vi "Calculate Position Orientation.vi"(8 "error in":errorcluster, 10 "Measured Global Positions":refnum<class "Vec3d Class.lvclass">[](array[class]), 11 "Known Local Positions":refnum<class "Vec3d Class.lvclass">[](array[class])) -> (0 "error out":errorcluster, 1 "Residual":dbl, 3 "PositionOrientation":T1)   [LabVIEW 2011]
uses:
  Vec3d Class/Vec3d Class.lvclass
  Type Definitions/Position_Orientation.ctl
  Orient3d Class/Orient3d Class.lvclass
  <vilib>/Analysis/_algsub.llb/Vector Norm Type.ctl
  <vilib>/Analysis/baseanly.llb/Real A x B.vi
  <vilib>/Analysis/_algsub.llb/Real Vector Norm.vi
  <vilib>/Analysis/7linalg.llb/Real Matrix Power.vi
  <vilib>/Analysis/Matrix/Numeric/Add/Add - RM,RM.vi
  <vilib>/Analysis/NI_AALBase.lvlib
  <vilib>/Analysis/NI_AALPro.lvlib
  <vilib>/Analysis/Matrix/NI_Matrix.lvlib
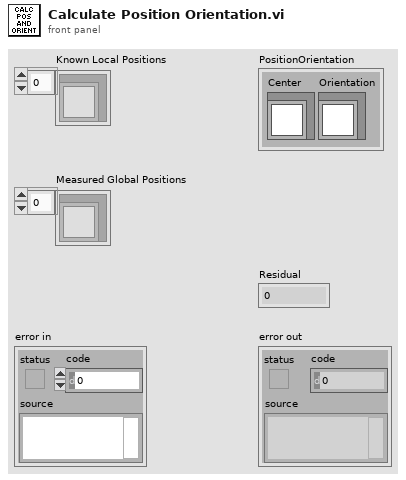
[diagram p1: front panel]
types:
  T1 = typedef "Position_Orientation.ctl" = cluster{"Center":refnum<class "Vec3d Class.lvclass">, "Orientation":refnum<class "Orient3d Class.lvclass">}
  T2 = typedef "NI_AALPro.lvlib/Vector Norm Type.ctl" = u16
  T3 = typedef "NI_Matrix.lvlib/RealMatrix.ctl" = dbl[][]
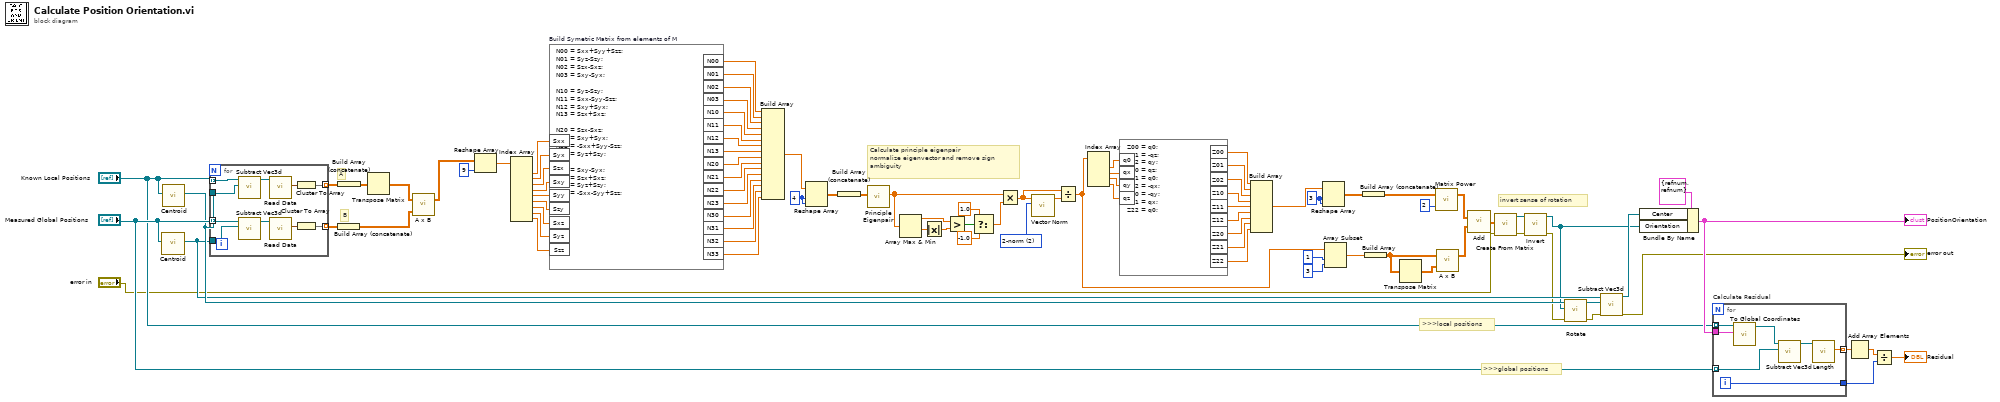
[diagram p0: block diagram]
diagram:
  w11 = 3 ("dimension size")
  w27 = 4 ("dimension size")
  w72 = T2 2 items=["1-norm"=1, "2-norm"=2, "Inf-norm"=3, "-Inf-norm"=4, "User Defined"=5] ("norm type")
  # "invert sense of rotation"
  # ">>>local positions"
  # ">>>global positions"
  # "Calculate principle eigenpair\nnormalize eigenvector and remove sign\nambiguity"
  # "B"
  # "A"
  n1 = call "Centroid.vi"("Points"="Measured Global Positions") -> ("Centroid"=w61:refnum<class "Vec3d Class.lvclass">)  [unwired: 10 in]
  n2 = call "Centroid.vi"("Points"="Known Local Positions") -> ("Centroid"=w62:refnum<class "Vec3d Class.lvclass">)  [unwired: 10 in]
  n3 = for {
    tunnel: "Known Local Positions" -> [w104] mode=indexing
    tunnel: "Measured Global Positions" -> [w102] mode=indexing
    tunnel: w61 -> [w101]
    tunnel: w62 -> [w103]
    tunnel: [w96] -> w86 mode=indexing
    tunnel: [w95] -> w85 mode=indexing
    n4 = call "Subtract Vec3d.vi"("Vec3d in 2"=w103, "Vec3d in 1"=w104) -> ("Vec3d Class out"=w100:refnum<class "Vec3d Class.lvclass">)  [unwired: 8 in, 1 out]
    n5 = call "Subtract Vec3d.vi"("Vec3d in 2"=w101, "Vec3d in 1"=w102) -> ("Vec3d Class out"=w97:refnum<class "Vec3d Class.lvclass">)  [unwired: 8 in, 1 out]
    n6 = call-dynamic "Read Data.vi"("Vec3d Class in"=w100) -> ("Data"=w99:cluster{"X":dbl, "Y":dbl, "Z":dbl})  [unwired: 8 in, 2 out]
    n7 = call-dynamic "Read Data.vi"("Vec3d Class in"=w97) -> ("Data"=w98:cluster{"X":dbl, "Y":dbl, "Z":dbl})  [unwired: 8 in, 2 out]
    n8 = Cluster To Array(cluster=w99) -> (array=w96:dbl[])
    n9 = Cluster To Array(cluster=w98) -> (array=w95:dbl[])
  }
  n10 = Build Array (concatenate)(w85) -> (w82:T3)
  n11 = Build Array (concatenate)(w86) -> (w84:T3)
  n12 = Transpose Matrix(1:w84) -> (0:w83:T3)
  n13 = call-poly <vilib>:"A x B.vi"("B"=w82, "A"=w83) -> ("A x B"=w56:T3)  [unwired: 1 out]
  n14 = Reshape Array(w56, 9 ("dimension size")) -> (w54:dbl[])
  n15 = Index Array(array=w54) -> (element #1=w53:dbl, element #2=w52:dbl, element #3=w51:dbl, element #4=w50:dbl, element #5=w49:dbl, element #6=w48:dbl, element #7=w47:dbl, element #8=w46:dbl, element #9=w45:dbl)  [unwired: 9 in]
  n16 = formula code="N00 = Sxx+Syy+Szz;\nN01 = Syz-Szy;\nN02 = Szx-Sxz;\nN03 = Sxy-Syx;\n\nN10 = Syz-Szy;\nN11 = Sxx-Syy-Szz;\nN12 = Sxy+Syx;\nN13 = Szx+Sxz;\n\nN20 = Szx-Sxz;\nN21 = Sxy+Syx;\nN22 = -Sxx+Syy-Szz;\nN23 = Syz+Szy;\n\nN30 = Sxy-Syx;\nN31 = Szx+Sxz;\nN32 = Syz+Szy;\nN33 = -Sxx-Syy+Szz;" "Build Symetric Matrix from elements of M"("Sxx"=w53, "Syx"=w52, "Szx"=w51, "Sxy"=w50, "Syy"=w49, "Szy"=w48, "Sxz"=w47, "Syz"=w46, "Szz"=w45) -> ("N00"=w44:dbl, "N01"=w43:dbl, "N02"=w42:dbl, "N03"=w41:dbl, "N10"=w40:dbl, "N11"=w39:dbl, "N12"=w38:dbl, "N13"=w37:dbl, "N20"=w36:dbl, "N21"=w35:dbl, "N22"=w34:dbl, "N23"=w33:dbl, "N30"=w32:dbl, "N31"=w31:dbl, "N32"=w30:dbl, "N33"=w29:dbl)
  n17 = Build Array(w44, w43, w42, w41, w40, w39, w38, w37, w36, w35, w34, w33, w32, w31, w30, w29) -> (w28:dbl[])
  n18 = Reshape Array(w28, w27, w27) -> (w26:dbl[][])
  n19 = Build Array (concatenate)(w26) -> (w81:T3)
  n20 = call "Principle Eigenpair.vi"("Matrix"=w81) -> ("Principal Eigenvector"=w73:dbl[])  [unwired: 9 in, 1 out]
  n21 = Array Max & Min(array=w73) -> (max value=w78:dbl, min value=w80:dbl)  [unwired: 2 out]
  n22 = Absolute Value(x=w80) -> (abs(x)=w79:dbl)
  n23 = Greater?(x=w78, y=w79) -> (0:w77:bool)
  n24 = Select(t=1.0, s=w77, f=-1.0) -> (s? t:f=w74:dbl)
  n25 = Multiply(x=w73, y=w74) -> (x*y=w70:dbl[])
  n26 = call-poly <vilib>:"Vector Norm.vi"("norm type"=w72, "Input Vector"=w70) -> ("norm"=w71:dbl)  [unwired: 8 in, 1 out]
  n27 = Divide(x=w70, y=w71) -> (x/y=w9:dbl[])
  n28 = Index Array(array=w9) -> (element #1=w25:dbl, element #2=w24:dbl, element #3=w23:dbl, element #4=w22:dbl)  [unwired: 4 in]
  n29 = formula code="Z00 = q0;\nZ01 = -qz;\nZ02 = qy;\nZ10 = qz;\nZ11 = q0;\nZ12 = -qx;\nZ20 = -qy;\nZ21 = qx;\nZ22 = q0;"("q0"=w25, "qx"=w24, "qy"=w23, "qz"=w22) -> ("Z00"=w21:dbl, "Z01"=w20:dbl, "Z02"=w19:dbl, "Z10"=w18:dbl, "Z11"=w17:dbl, "Z12"=w16:dbl, "Z20"=w15:dbl, "Z21"=w14:dbl, "Z22"=w13:dbl)
  n30 = Build Array(w21, w20, w19, w18, w17, w16, w15, w14, w13) -> (w12:dbl[])
  n31 = Reshape Array(w12, w11, w11) -> (w10:dbl[][])
  n32 = Array Subset(array=w9, index=1, length=3) -> (w8:dbl[])
  n33 = Build Array (concatenate)(w10) -> (w67:T3)
  n34 = Build Array(w8) -> (w69:T3)
  n35 = Transpose Matrix(1:w69) -> (0:w68:T3)
  n36 = call-poly <vilib>:"Matrix Power.vi"("n"=2, "Input Matrix"=w67) -> ("Matrix Power"=w64:T3)  [unwired: 1 out]
  n37 = call-poly <vilib>:"A x B.vi"("B"=w68, "A"=w69) -> ("A x B"=w65:T3)  [unwired: 1 out]
  n38 = call-poly <vilib>:"Add.vi"("Real Matrix B"=w65, "Real Matrix A"=w64) -> ("A + B"=w63:T3)
  n39 = call "Create From Matrix.vi"("error in"="error in", "Rotation Matrix"=w63) -> ("error out"=w3:errorcluster, "Orient3d out"=w4:refnum<class "Orient3d Class.lvclass">)  [unwired: 8 in]
  n40 = call "Invert.vi"("error in"=w3, "Orient3d in"=w4) -> ("error out"=w1:errorcluster, "Orient3d out"=w2:refnum<class "Orient3d Class.lvclass">)  [unwired: 8 in]
  n41 = call-dynamic "Rotate.vi"("error in"=w1, "Orient3d in"=w2, "Vec3d in"=w62) -> ("error out"=w58:errorcluster, "Vec3d out"=w60:refnum<class "Vec3d Class.lvclass">)  [unwired: 7 in]
  n42 = call "Subtract Vec3d.vi"("error in (no error)"=w58, "Vec3d in 2"=w60, "Vec3d in 1"=w61) -> ("error out"=→"error out":errorcluster, "Vec3d Class out"=w59:refnum<class "Vec3d Class.lvclass">)  [unwired: 7 in]
  n43 = Bundle By Name(cluster=T1 {"Center"=refnum, "Orientation"=refnum} ("Center/Orientation"), "Center"=w59, "Orientation"=w2) -> (w93:T1)
  "PositionOrientation" <- w93
  n44 = for "Calculate Residual" {
    tunnel: "Known Local Positions" -> [w111] mode=indexing
    tunnel: "Measured Global Positions" -> [w109] mode=indexing
    tunnel: w93 -> [w110]
    tunnel: [w106] -> w90
    tunnel: [w105] -> w92 mode=indexing
    i -> [w106]
    n45 = call "To Global Coordinates.vi"("Center/Orientation"=w110, "Local Coordinates"=w111) -> ("Global Coordinates"=w108:refnum<class "Vec3d Class.lvclass">)  [unwired: 8 in, 1 out]
    n46 = call "Subtract Vec3d.vi"("Vec3d in 2"=w109, "Vec3d in 1"=w108) -> ("Vec3d Class out"=w107:refnum<class "Vec3d Class.lvclass">)  [unwired: 8 in, 1 out]
    n47 = call-dynamic "Length.vi"("Vec3d in"=w107) -> ("Length"=w105:dbl)  [unwired: 8 in, 2 out]
  }
  n48 = Add Array Elements(numeric array=w92) -> (sum=w91:dbl)
  n49 = Divide(x=w91, y=w90) -> (x/y=→"Residual":dbl)
